vi "save_VI.vi"() -> ()   [LabVIEW 2020]
panel:
  out "error out":errorcluster
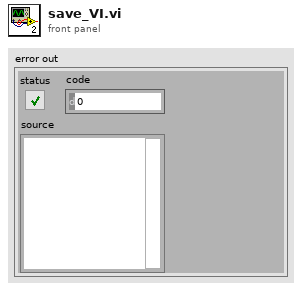
[diagram p1: front panel]
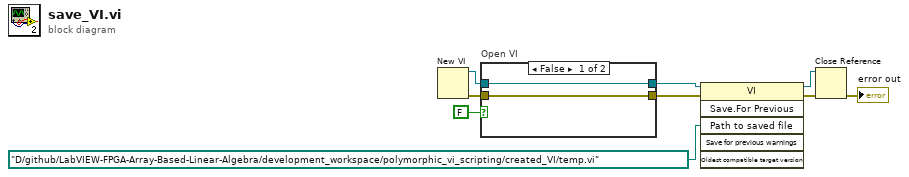
[diagram p0: block diagram]
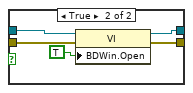
[diagram p2: hidden frame]
diagram:
  n1 = New VI() -> (0:w8:errorcluster, 3:w9:refnum<vi>)  [unwired: 7 in]
  n2 = case "Open VI" shown="False" FALSE {
    tunnel: w9 -> [w10 w16]
    tunnel: w8 -> [w11 w15]
    tunnel: [w10 w13] -> w7
    tunnel: [w11 w12] -> w6
    frame False {
    }
    frame True {
      n3 = property class="VI"(reference=w16, error in=w15, "BDWin.Open"=TRUE ("Block Diagram Window:Open")) -> (reference out=w13:refnum<vi>, error out=w12:errorcluster)
    }
  }
  n4 = invoke class="VI" method="Save.For Previous"(reference=w7, error in=w6, "Path to saved file"=path "D:/github/LabVIEW-FPGA-Array-Based-Linear-Algebra/development_workspace/polymorphic_vi_scripting/created_VI/temp.vi" ("Path to Saved File")) -> (reference out=w5:refnum<vi>, error out=w4:errorcluster)  [unwired: 3 in, 4 out]
  n5 = Close Reference(reference=w5, error in (no error)=w4) -> (error out=→"error out":errorcluster)
